vi "Read SA Pin.vi"(8 "error in (no error)":errorcluster, 11 "GSM_PVT in":refnum<class "GSM_PVT.lvclass">=refnum) -> (0 "error out":errorcluster, 2 "SA Pin":string, 3 "GSM_PVT out":refnum<class "GSM_PVT.lvclass">)   [LabVIEW 2016, in "SeqAuto Evaluations.lvlib" / "GSM_PVT.lvclass"]
uses:
  GSM_PVT.lvclass
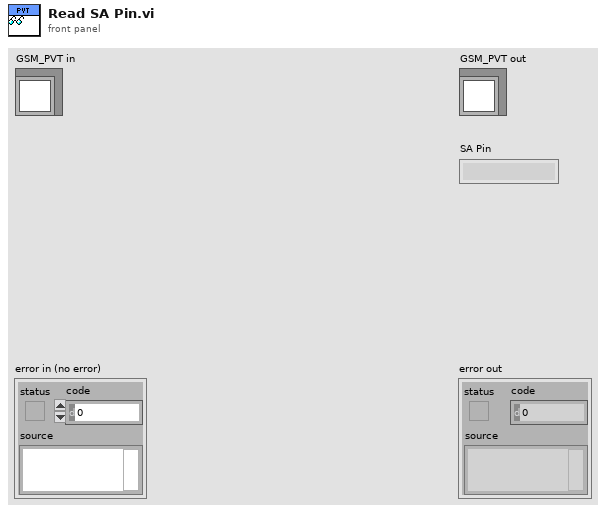
[diagram p1: front panel]
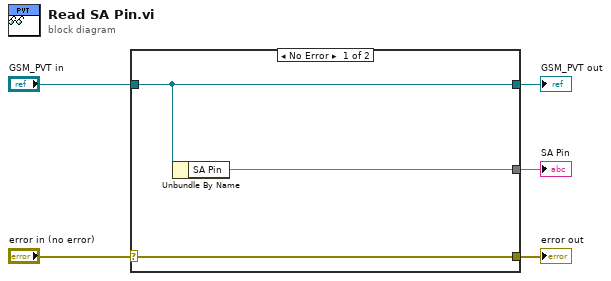
[diagram p0: block diagram]
diagram:
  n1 = case shown="No Error" "error in (no error)" {
    selector: "error in (no error)" -> [w8 w9]
    tunnel: [w8 w9] -> w4
    tunnel: [w7 w10] -> w2
    tunnel: "GSM_PVT in" -> [w7 w10]
    tunnel: [w6 _] -> w1
    frame No Error {
      n2 = Unbundle By Name(w7) -> ("SA Pin"=w6)
    }
    frame Error {
    }
  }
  "error out" <- w4
  "GSM_PVT out" <- w2
  "SA Pin" <- w1
